vi "Cache_Members Global_Write.vi"(10 "Member Map":T1, 11 "Class Name":string) -> ()   [LabVIEW 2019, in "ClassLoader.lvlib"]
uses:
  ClassLoader.lvlib
  Cache_Members Global.vi
  <vilib>/Utility/Data Type/Member VI Info.ctl
  Ctl/Ctl_Member Map.ctl
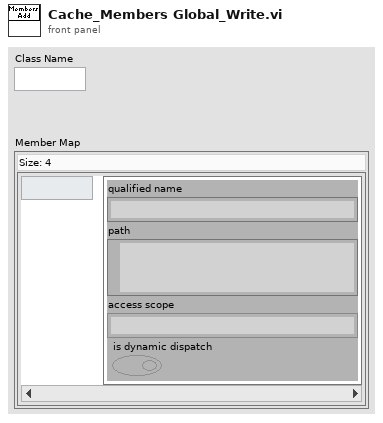
[diagram p1: front panel]
types:
  T1 = typedef "ClassLoader.lvlib/Ctl_Member Map.ctl" = map{string, T2}
  T2 = typedef "Member VI Info.ctl" = cluster{"qualified name":string, "path":path, "access scope":enum32{"invalid scope", "public", "private", "protected", "community"}, "is dynamic dispatch":bool}
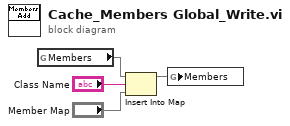
[diagram p0: block diagram]
diagram:
  n1 = global read "Cache_Members Global.vi" "Members"() -> (w2:map{string, T1})
  n2 = Insert Into Map(map in=w2, key="Class Name", value="Member Map") -> (map out=w3:map{string, T1})  [unwired: 2 out]
  n3 = global write "Cache_Members Global.vi" "Members"(w3) -> ()
